vi "estadoGeneradores.vi"() -> ()   [LabVIEW 2018]
panel:
  in  "estado G6":string
  in  "estado G5":string
  in  "estado G4":string
  in  "estado G3":string
  in  "estado G2":string
  in  "estado G1":string
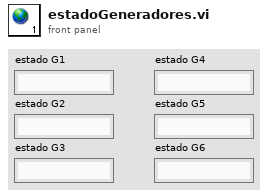
[diagram p1: front panel]
diagram:
